vi "CLD 16 state machine front panel.vi"() -> ()   [LabVIEW 2009]
doc: "CLD 16 Exercise"
uses:
  CLD 16 Control Panel.ctl
  CLD 16 Status Panel.ctl
panel:
  in  "Stop Button":bool
  out "Line Two Active":bool
  out "Line One Active":bool
  in  "Control Panel Two":T1
  out "Process Control":T2 {"Process Value" format="%#.3g"}
  in  "Control Panel One":T1
  # "Display Panel"
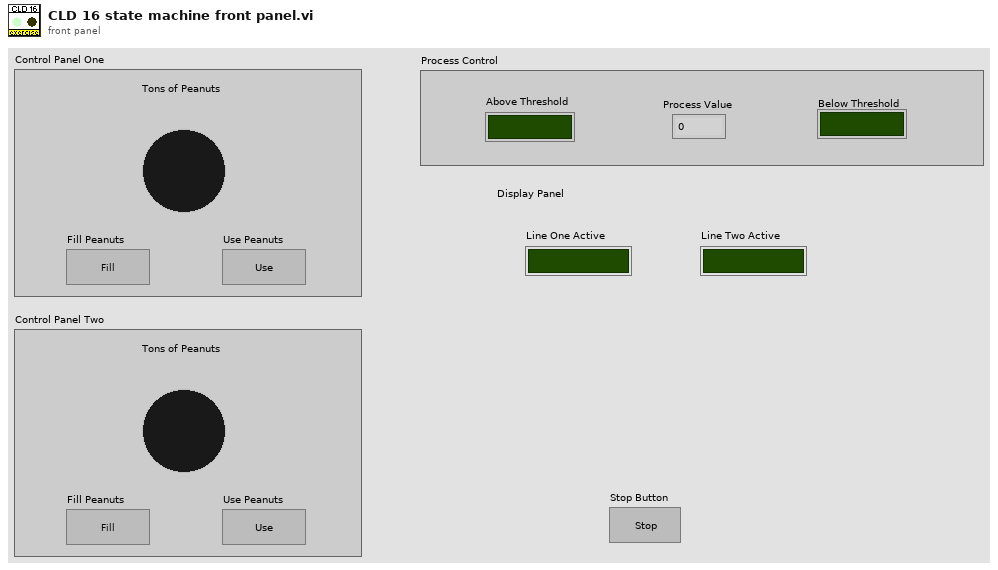
[diagram p1: front panel]
types:
  T1 = typedef "CLD 16 Control Panel.ctl" = cluster{"Tons of Peanuts":i8, "Fill Peanuts":bool, "Use Peanuts":bool}
  T2 = typedef "CLD 16 Status Panel.ctl" = cluster{"Above Threshold":bool, "Below Threshold":bool, "Process Value":dbl}
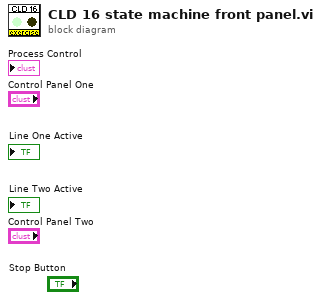
[diagram p0: block diagram]
diagram:
